vi "Final Tilt Platform Controller.vi"() -> ()   [LabVIEW 2015]
uses:
  Control 1.ctl
  <vilib>/DAQmx/read.llb/DAQmx Read (Analog 1D Wfm NChan NSamp).vi
  <vilib>/DAQmx/read.llb/DAQmx Read (Digital Wfm 1Chan NSamp).vi
  <vilib>/DAQmx/write.llb/DAQmx Write (Digital 1D Bool 1Chan 1Samp).vi
  <vilib>/Utility/file.llb/Read From Spreadsheet File (DBL).vi
  <vilib>/Utility/file.llb/Read Delimited Spreadsheet (DBL).vi
  <vilib>/Utility/file.llb/Write Delimited Spreadsheet (DBL).vi
  <vilib>/DAQmx/create/channels.llb/DAQmx Create Channel (DO-Digital Output).vi
  <vilib>/DAQmx/create/channels.llb/DAQmx Create Channel (AI-Voltage-Basic).vi
  <vilib>/DAQmx/configure/timing.llb/DAQmx Timing (Sample Clock).vi
  <vilib>/DAQmx/configure/trigger.llb/DAQmx Start Trigger (Digital Edge).vi
  <vilib>/DAQmx/create/channels.llb/DAQmx Create Channel (DI-Digital Input).vi
  <vilib>/DAQmx/create/channels.llb/DAQmx Create Channel (CO-Pulse Generation-Ticks).vi
  <vilib>/DAQmx/configure/timing.llb/DAQmx Timing (Implicit).vi
  <vilib>/DAQmx/miscellaneous.llb/DAQmx Fill In Error Info.vi
  <vilib>/Waveform/DTblOps.llb/DTbl Digital to Boolean Array.vi
panel:
  out "incl":dbl[](array[numeric])
  in  "Start from Tilt":i32=1
  out "Ready":bool
  in  "Replay File":path
  in  "Load Sequence":bool
  in  "Format":string="%.3f"
  in  "Delimiter":string=","
  in  "Column/Row Major":bool
  in  "Append to File?":bool=TRUE
  out "File Path":path
  out "Waveform Chart (Multiple Plots)":dbl[][](graph)
  in  "Callib Acce":bool
  in  "Callib Load Cell":bool
  in  "Transect?":bool
  in  "Week Number":dbl
  in  "Rat ID":string
  out "4":bool
  out "5":bool
  out "6":bool
  out "2":bool
  out "1":bool
  out "3":bool
  in  "Baseline Angle":dbl
  out "Angle":i32
  out "Total Force (g)":i32
  out "Completed Tilts":i32
  out "Current Tilt":i32
  out "Current ITI (s)":i32
  in  "Tirgger 6":bool=TRUE
  in  "Enable Left Slow":bool=TRUE
  in  "Enable Left Medium":bool=TRUE
  in  "Enable Left Fast":bool=TRUE
  in  "Enable Right Slow":bool=TRUE
  in  "Enable Right Medium":bool=TRUE
  in  "Enable Right Fast":bool=TRUE
  out "Left Slow":i32
  out "Left Medium":i32
  out "Left Fast":i32
  out "Right Slow":i32
  out "Right Medium":i32
  out "Right Fast":i32
  out "Practice?":bool
  in  "Stop 2":bool
  in  "Pause":bool=TRUE
  in  "Start":bool
  in  "Trial Per Tilt":T1=100.0
  in  "ITI Base (s)":dbl=2.0 format="%#.2g"
  in  "ITI Random Multiplier":dbl=1.0 format="%#.2g"
  in  "Clock Source":i32(slide)=1 caption="Choose a setting:" scale=0.0..1.0
  # "Rat Ground Reaction Forces"
  # "Clock Source"
  # "Tilt Parameters"
  # "Enable"
  # "Animal Info"
  # "Right"
  # "Left"
  # "Current Values"
  # "Enable"
  # "Callibration"
  # "File Information"
  # "Replay Sequence"
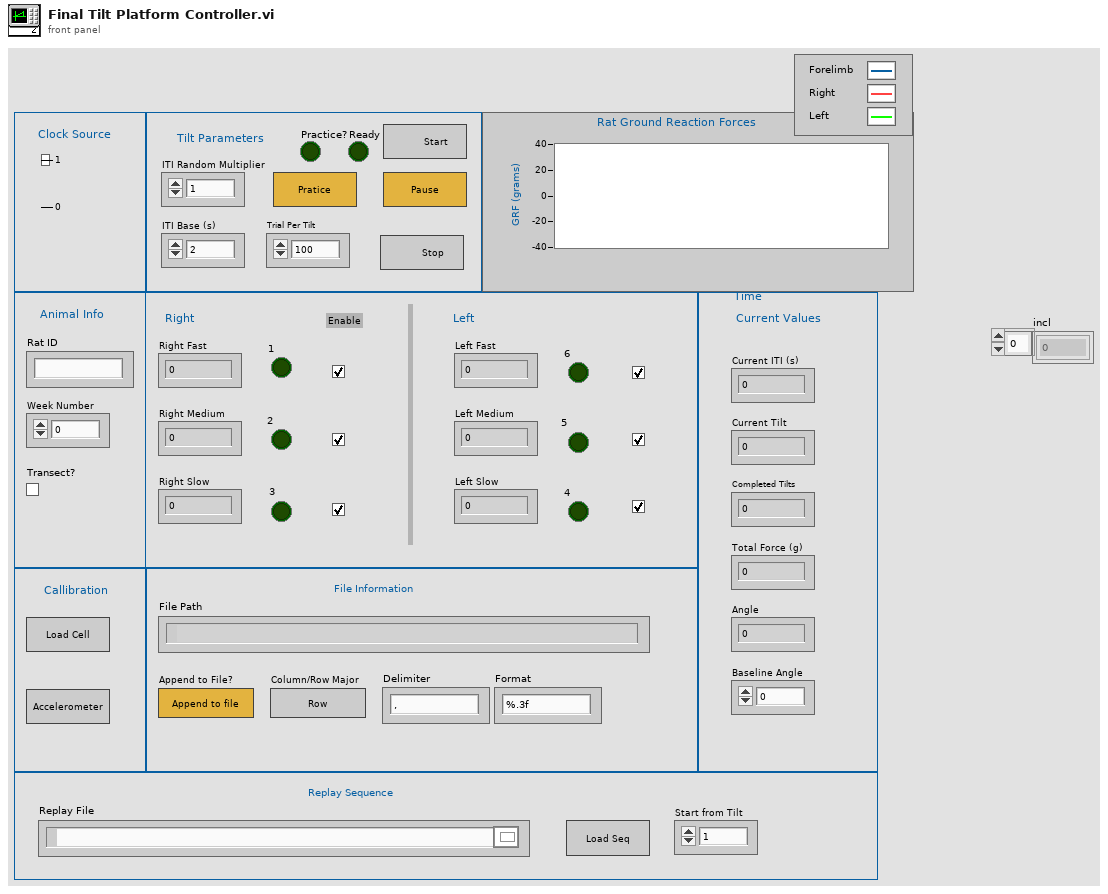
[diagram p1: front panel]
types:
  T1 = typedef "Control 1.ctl" = dbl
  T2 = enum16{"open", "replace", "create", "open or create", "replace or create", "replace or create with confirmation"}
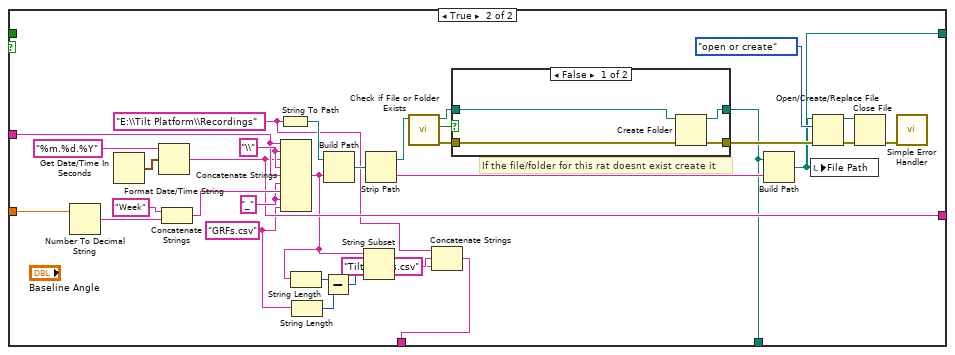
[diagram p2: hidden frame]
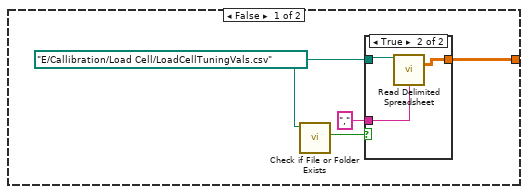
[diagram p4: hidden frame]
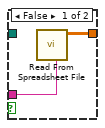
[diagram p5: hidden frame]
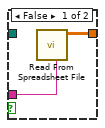
[diagram p6: hidden frame]
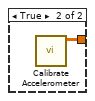
[diagram p7: hidden frame]
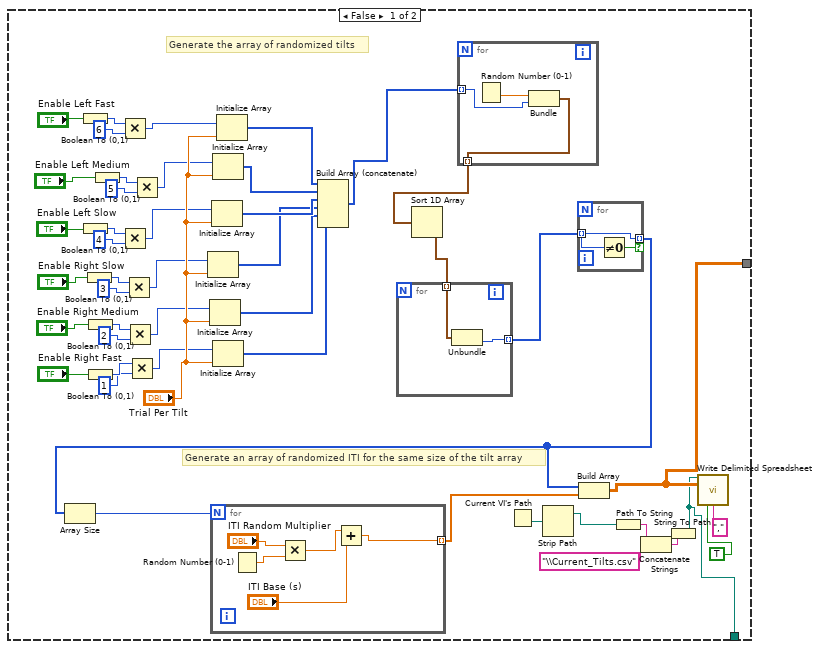
[diagram p8: hidden frame]
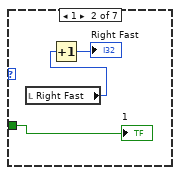
[diagram p12: hidden frame]
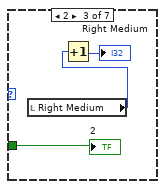
[diagram p13: hidden frame]
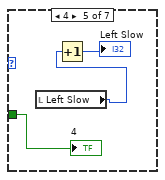
[diagram p14: hidden frame]
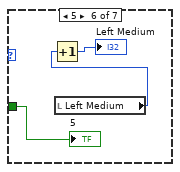
[diagram p15: hidden frame]
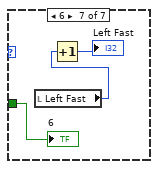
[diagram p16: hidden frame]
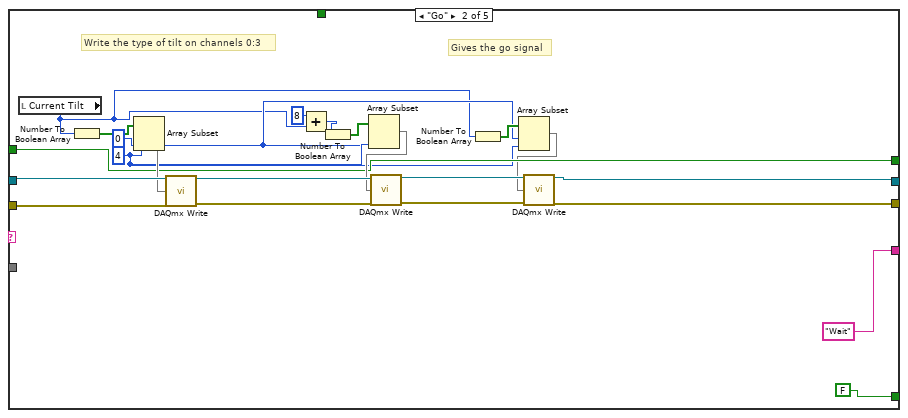
[diagram p17: hidden frame]
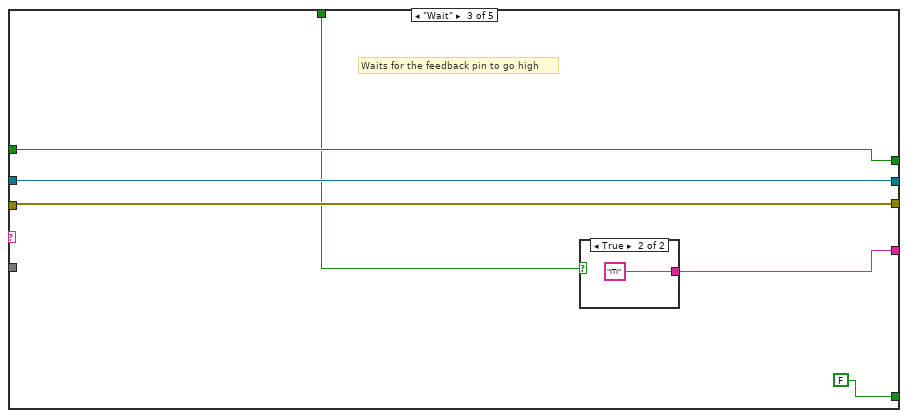
[diagram p18: hidden frame]
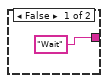
[diagram p19: hidden frame]
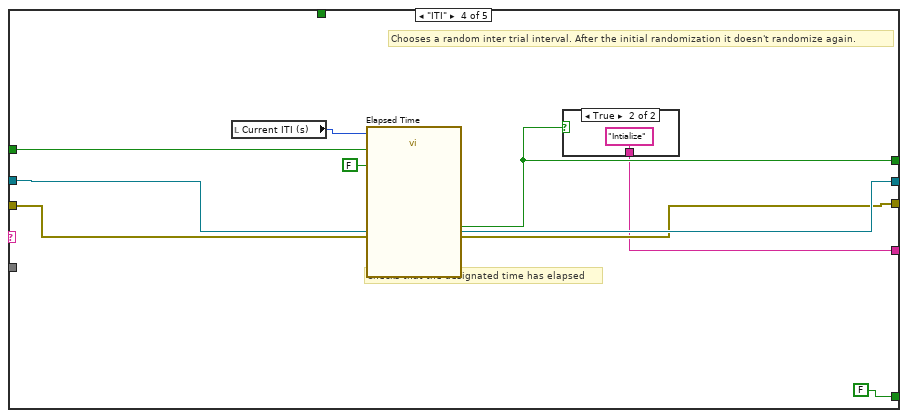
[diagram p20: hidden frame]
diagram:
  # "DataCol/KEY\n1-ai4 (17)=forelimb GRF\n2-ai5 (20)=RHL GRF\n3-ai6 (25)=LHL GRF\n4-ai0=ACC1\n5-ai1=ACC2\n6-ai2=ACC3\n7-ai3=inclinometer"
  # "The GUI these items are not touched. Only through local variables"
  n1 = flat-sequence {
    tunnel: ["Tirgger 6"] -> w70
    tunnel: [w80] -> w69
    tunnel: [w76] -> w63
    tunnel: [w74] -> w15
    tunnel: [w73] -> w8
    tunnel: [w72] -> w1
    tunnel: w70 -> [w127]
    tunnel: [w127] -> w68
    tunnel: w69 -> [w126]
    tunnel: [w126] -> w67
    tunnel: w63 -> [w125]
    tunnel: [w125] -> w62
    tunnel: [w123] -> w30
    tunnel: [w122] -> w16
    tunnel: w15 -> [w122]
    tunnel: [w121] -> w9
    tunnel: w8 -> [w121]
    tunnel: [w120] -> w2
    tunnel: w1 -> [w120]
    tunnel: w68 -> [w146]
    tunnel: [w146] -> w51
    tunnel: [w145] -> w49
    tunnel: w67 -> [w145]
    tunnel: [w144] -> w47
    tunnel: w62 -> [w144]
    tunnel: [w143] -> w31
    tunnel: w30 -> [w143]
    tunnel: [w141] -> w27
    tunnel: [w140] -> w17
    tunnel: w16 -> [w140]
    tunnel: [w139] -> w10
    tunnel: w9 -> [w139]
    tunnel: [w138] -> w3
    tunnel: w2 -> [w138]
    tunnel: w51 -> [w164]
    tunnel: [w164] -> w50
    tunnel: w49 -> [w163]
    tunnel: [w163] -> w48
    tunnel: w47 -> [w162]
    tunnel: [w162] -> w46
    tunnel: [w161] -> w32
    tunnel: w31 -> [w161]
    tunnel: [w160] -> w28
    tunnel: w27 -> [w160]
    tunnel: [w159] -> w18
    tunnel: w17 -> [w159]
    tunnel: [w158] -> w11
    tunnel: w10 -> [w158]
    tunnel: [w157] -> w4
    tunnel: w3 -> [w157]
    tunnel: w50 -> [w175]
    tunnel: [w175] -> w61
    tunnel: w48 -> [w174]
    tunnel: [w174] -> w60
    tunnel: w46 -> [w173]
    tunnel: [w173] -> w59
    tunnel: [w171] -> w45
    tunnel: [w170] -> w33
    tunnel: w32 -> [w170]
    tunnel: w28 -> [w169]
    tunnel: [w169] -> w26
    tunnel: [w168] -> w22
    tunnel: [w167] -> w19
    tunnel: w18 -> [w167]
    tunnel: [w166] -> w12
    tunnel: w11 -> [w166]
    tunnel: [w165] -> w5
    tunnel: w4 -> [w165]
    tunnel: [w301] -> w66
    tunnel: w61 -> [_]
    tunnel: [w294] -> w65
    tunnel: [w293] -> w64
    tunnel: w60 -> [w250]
    tunnel: w59 -> [_]
    tunnel: [w284] -> w58
    tunnel: [w283] -> w57
    tunnel: [w280] -> w52
    tunnel: w45 -> [w279]
    tunnel: [w279] -> w44
    tunnel: [w276] -> w43
    tunnel: [w275] -> w42
    tunnel: [w259] -> w39
    tunnel: [w258] -> w38
    tunnel: w33 -> [w252]
    tunnel: [w252] -> w29
    tunnel: w26 -> [w251]
    tunnel: [w251] -> w25
    tunnel: [w248] -> w23
    tunnel: w22 -> [w248]
    tunnel: [w247] -> w20
    tunnel: w19 -> [w247]
    tunnel: [w246] -> w13
    tunnel: w12 -> [w246]
    tunnel: [w245] -> w6
    tunnel: w5 -> [w245]
    tunnel: w66 -> [w340]
    tunnel: w65 -> [w339]
    tunnel: w64 -> [w337]
    tunnel: w58 -> [w342]
    tunnel: w57 -> [w341]
    tunnel: [w338] -> w56
    tunnel: [w336] -> w55
    tunnel: [w335] -> w54
    tunnel: [w334] -> w53
    tunnel: w52 -> [w332]
    tunnel: w44 -> [w331]
    tunnel: w43 -> [w330]
    tunnel: w42 -> [w329]
    tunnel: [w328] -> w41
    tunnel: [w327] -> w40
    tunnel: w39 -> [w325]
    tunnel: w38 -> [w326]
    tunnel: [w323] -> w37
    tunnel: [w324] -> w36
    tunnel: [w321] -> w35
    tunnel: [w320] -> w34
    tunnel: w29 -> [w319]
    tunnel: w25 -> [w318]
    tunnel: [w317] -> w24
    tunnel: w23 -> [w317]
    tunnel: [w316] -> w21
    tunnel: w20 -> [w316]
    tunnel: [w315] -> w14
    tunnel: w13 -> [w315]
    tunnel: [w314] -> w7
    tunnel: w6 -> [w314]
    tunnel: w56 -> [w522]
    tunnel: w55 -> [w521]
    tunnel: w54 -> [w520]
    tunnel: w53 -> [w519]
    tunnel: w41 -> [w517]
    tunnel: w40 -> [w518]
    tunnel: w37 -> [w512]
    tunnel: w36 -> [w513]
    tunnel: w35 -> [_]
    tunnel: w34 -> [_]
    tunnel: w24 -> [w511]
    tunnel: w21 -> [w510]
    tunnel: w14 -> [w509]
    tunnel: w7 -> [w508]
    frame #0 {
      # "This keeps the program frozen until you hit start. This way it gives you time to change anything you need to update for the tilt types"
      # "Determine if this is a practice session. Causes files not to be saved"
      n2 = while {
        stop <- "Start" stop-if-true
      }
    }
    frame #1 {
      # "If the file doesnt exist create it"
      # "Save the file"
      # "If it's not a practice"
      n3 = Not(x="Tirgger 6") -> (.not. x?=w73:bool)
      n4 = local write "Practice?"("Tirgger 6") -> ()
      n5 = case shown="False" w73 {
        tunnel: "Transect?" -> [_ _]
        tunnel: "Week Number" -> [_ w95]
        tunnel: "Rat ID" -> [_ w94]
        tunnel: [_ w91] -> w80
        tunnel: [_ w93] -> w76
        tunnel: [_ w83] -> w74
        tunnel: [_ w81] -> w72
        frame False {
        }
        frame True {
          w96 = "_"
          w99 = "\\" ("string")
          w84 = "E:\\Tilt Platform\\Recordings"
          w87 = "GRFs.csv" ("string")
          # "If the file/folder for this rat doesnt exist create it"
          n6 = Number To Decimal String(number=w95) -> (decimal integer string=w112:string)  [unwired: 1 in]
          n7 = Get Date/Time In Seconds() -> (seconds since 1Jan1904=w110:timestamp)
          n8 = Format Date/Time String(time format string (%c)="%m.%d.%Y", seconds (now)=w110) -> (date/time string=w93:string)  [unwired: 1 in]
          n9 = Concatenate Strings("Week" ("string"), w112) -> (w98:string)
          n10 = String To Path(string=w84) -> (path=w111:path)
          n11 = Concatenate Strings(w94, w99, w93, w99, w94, w96, w98, w96, w87) -> (w90:string)
          n12 = String Length(string=w90) -> (length=w89:i32)
          n13 = String Length(string=w87) -> (length=w88:i32)
          n14 = Subtract(x=w89, y=w88) -> (x-y=w86:i32)
          n15 = Build Path(base path=w111, name or relative path=w90) -> (appended path=w108:path)
          n16 = String Subset(string=w90, length (rest)=w86) -> (substring=w85:string)  [unwired: 1 in]
          n17 = Strip Path(path=w108) -> (stripped path=w107:path, name=w97:string)
          n18 = call <vilib>:"Check if File or Folder Exists.vi"("path"=w107) -> ("error out"=w105:errorcluster, "file or folder exists?"=w106:bool, "dup path"=w92:path)  [unwired: 8 in]
          n19 = Concatenate Strings(w84, w85, "Tilt_Types.csv" ("string")) -> (w83:string)
          n20 = case shown="False" w106 {
            tunnel: w92 -> [w117 w119]
            tunnel: w105 -> [w116 w118]
            tunnel: [w115 w119] -> w81
            tunnel: [w114 w118] -> w102
            frame False {
              n21 = Create Folder(path (use dialog)=w117, error in=w116) -> (created path=w115:path, error out=w114:errorcluster)  [unwired: 1 in, 1 out]
            }
            frame True {
            }
          }
          n22 = Build Path(base path=w81, name or relative path=w97) -> (appended path=w91:path)
          n23 = local write "File Path"(w91) -> ()
          n24 = Open/Create/Replace File(file path (use dialog)=w91, error in=w102, operation (0:open)=T2."open or create") -> (refnum out=w104:refnum<file>, error out=w101:errorcluster)  [unwired: 3 in, 1 out]
          n25 = Close File(refnum=w104, error in=w101) -> (error out=w100:errorcluster)  [unwired: 1 out]
          n26 = call <vilib>:"Simple Error Handler.vi"("error in (no error)"=w100) -> ()  [unwired: 4 in, 5 out]
        }
      }
    }
    frame #2 {
      # "Otherwise load the previous callibration values"
      # "Pull up sub vi"
      # "If you chose to calibrate the load cells"
      n27 = case shown="True" "Callib Load Cell" {
        tunnel: [w129 w137] -> w123
        frame False {
          w130 = path "E:/Callibration/Load Cell/LoadCellTuningVals.csv" ("file path (dialog if empty)")
          n28 = call <vilib>:"Check if File or Folder Exists.vi"("path"=w130) -> ("file or folder exists?"=w131:bool)  [unwired: 8 in, 2 out]
          n29 = case shown="True" w131 {
            tunnel: w130 -> [_ w135]
            tunnel: [w133 w134] -> w129
            tunnel: "," ("delimiter (\\t)") -> [w132 w136]
            frame False {
              n30 = call-poly <vilib>:"Read From Spreadsheet File.vi"("delimiter (\\t)"=w132) -> ("all rows"=w133:dbl[][])  [unwired: 6 in, 4 out]
            }
            frame True {
              n31 = call-poly <vilib>:"Read Delimited Spreadsheet.vi"("file path (dialog if empty)"=w135, "delimiter (\\t)"=w136) -> ("all rows"=w134:dbl[][])  [unwired: 8 in, 5 out]
            }
          }
        }
        frame True {
          n32 = call "Calibrate load cells.vi"() -> ("Slope and Intercept"=w137:dbl[][])  [unwired: 11 in]
        }
      }
    }
    frame #3 {
      # "Otherwise load the previous values"
      # "Load the sub vi"
      # "If you chose to calibrate the accelerometer"
      n33 = case shown="False" "Callib Acce" {
        tunnel: [w149 w156] -> w141
        frame False {
          w148 = path "E:/Callibration/Accelerometer/AccTuningVals.csv" ("file path (dialog if empty)")
          n34 = call <vilib>:"Check if File or Folder Exists.vi"("path"=w148) -> ("file or folder exists?"=w147:bool)  [unwired: 8 in, 2 out]
          n35 = case shown="True" w147 {
            tunnel: "," ("delimiter (\\t)") -> [w151 w155]
            tunnel: [w152 w154] -> w149
            tunnel: w148 -> [_ w153]
            frame False {
              n36 = call-poly <vilib>:"Read From Spreadsheet File.vi"("delimiter (\\t)"=w151) -> ("all rows"=w152:dbl[][])  [unwired: 6 in, 4 out]
            }
            frame True {
              n37 = call-poly <vilib>:"Read Delimited Spreadsheet.vi"("file path (dialog if empty)"=w153, "delimiter (\\t)"=w155) -> ("all rows"=w154:dbl[][])  [unwired: 8 in, 5 out]
            }
          }
        }
        frame True {
          n38 = call "Calibrate Accelerometer.vi"() -> ("Output"=w156:dbl[][])  [unwired: 9 in]
        }
      }
    }
    frame #4 {
    }
    frame #5 {
      # "Is this a practice session?"
      # "load cell regression params"
      # "acceleremeter regression params"
      n39 = case shown="True" "Load Sequence" {
        tunnel: [w177 w235] -> w171
        tunnel: [w176 _] -> w168
        frame False {
          # "Generate an array of randomized ITI for the same size of the tilt array"
          # "Generate the array of randomized tilts"
          n40 = Boolean To (0,1)(Boolean="Enable Left Fast") -> (0, 1=w219:i16)
          n41 = Boolean To (0,1)(Boolean="Enable Left Slow") -> (0, 1=w211:i16)
          n42 = Boolean To (0,1)(Boolean="Enable Right Slow") -> (0, 1=w208:i16)
          n43 = Boolean To (0,1)(Boolean="Enable Right Medium") -> (0, 1=w203:i16)
          n44 = Boolean To (0,1)(Boolean="Enable Right Fast") -> (0, 1=w199:i16)
          n45 = Boolean To (0,1)(Boolean="Enable Left Medium") -> (0, 1=w216:i16)
          n46 = Multiply(x=w219, y=6 ("length")) -> (x*y=w213:i32)
          n47 = Multiply(x=w211, y=4 ("length")) -> (x*y=w205:i32)
          n48 = Multiply(x=w208, y=3 ("length")) -> (x*y=w204:i32)
          n49 = Multiply(x=w203, y=2 ("length")) -> (x*y=w200:i32)
          n50 = Multiply(x=w199, y=1 ("length")) -> (x*y=w196:i32)
          n51 = Multiply(x=w216, y=5 ("length")) -> (x*y=w212:i32)
          n52 = Initialize Array(w204, "Trial Per Tilt") -> (w192:i32[])
          n53 = Initialize Array(w200, "Trial Per Tilt") -> (w191:i32[])
          n54 = Initialize Array(w205, "Trial Per Tilt") -> (w193:i32[])
          n55 = Initialize Array(w212, "Trial Per Tilt") -> (w194:i32[])
          n56 = Initialize Array(w196, "Trial Per Tilt") -> (w190:i32[])
          n57 = Initialize Array(w213, "Trial Per Tilt") -> (w195:i32[])
          n58 = Build Array (concatenate)(w195, w194, w193, w192, w191, w190) -> (w188:i32[])
          n59 = for {
            tunnel: w188 -> [w232] mode=indexing
            tunnel: [w233] -> w222 mode=indexing
            n60 = Random Number (0-1)() -> (number: 0 to 1=w234:dbl)
            n61 = Bundle("number: 0 to 1"=w234, w232) -> (w233:cluster{"number: 0 to 1":dbl, i32})  [unwired: 1 in]
          }
          n62 = Sort 1D Array(array=w222) -> (sorted array=w221:cluster{"number: 0 to 1":dbl, i32}[])
          n63 = for {
            tunnel: w221 -> [w231] mode=indexing
            tunnel: [w230] -> w189 mode=indexing
            n64 = Unbundle(w231) -> (w230:i32)  [unwired: 1 out]
          }
          n65 = Current VI's Path() -> (path=w184:path)
          n66 = Strip Path(path=w184) -> (stripped path=w183:path)  [unwired: 1 out]
          n67 = for {
            tunnel: [w228] -> w178 mode=indexing if=w229
            tunnel: w189 -> [w228] mode=indexing
            n68 = Not Equal To 0?(x=w228) -> (x != 0?=w229:bool)
          }
          n69 = Array Size(array=w178) -> (size(s)=w187:i32)
          n70 = for {
            N: w187 -> [_]
            tunnel: [w223] -> w186 mode=indexing
            n71 = Random Number (0-1)() -> (number: 0 to 1=w226:dbl)
            n72 = Multiply(x="ITI Random Multiplier", y=w226) -> (x*y=w225:dbl)
            n73 = Add(x=w225, y="ITI Base (s)") -> (x+y=w223:dbl)
          }
          n74 = Build Array(w178, w186) -> (w177:dbl[][])
          n75 = Path To String(path=w183) -> (string=w182:string)
          n76 = Concatenate Strings(w182, "\\Current_Tilts.csv") -> (w180:string)
          n77 = String To Path(string=w180) -> (path=w176:path)
          n78 = call-poly <vilib>:"Write Delimited Spreadsheet.vi"("file path (dialog if empty)"=w176, "2D data"=w177, "transpose? (F)"=TRUE ("transpose? (no:F)"), "delimiter (\\t)"="," ("delimiter (\\t)")) -> ()  [unwired: 10 in, 2 out]
        }
        frame True {
          n79 = Decrement(x="Start from Tilt") -> (x-1=w237:i32)
          n80 = call-poly <vilib>:"Read Delimited Spreadsheet.vi"("file path (dialog if empty)"="Replay File", "delimiter (\\t)"="," ("delimiter (\\t)")) -> ("all rows"=w242:dbl[][])  [unwired: 8 in, 5 out]
          n81 = Array Size(array=w242) -> (size(s)=w241:i32[])
          n82 = Array Max & Min(array=w241) -> (max value=w239:i32)  [unwired: 3 out]
          n83 = Subtract(x=w239, y=w237) -> (x-y=w240:i32)
          n84 = Array Subset(array=w242, index (row)=w237, length (row)=w240) -> (w236:dbl[][])  [unwired: 2 in]
          n85 = Transpose 2D Array(2D array=w236) -> (transposed array=w235:dbl[][])
        }
      }
    }
    frame #6 {
      w263 = 10214 items=["High"=10192, "Low"=10214] ("idle state")
      w262 = 10123 items=["Finite Samples"=10178, "Continuous Samples"=10123, "Hardware Timed Single Point"=12522] ("sample mode")
      w281 = 10123 items=["Finite Samples"=10178, "Continuous Samples"=10123, "Hardware Timed Single Point"=12522] ("sample mode")
      w295 = 10083 items=["default"=-1, "RSE"=10083, "NRSE"=10078, "Differential"=10106, "Pseudodifferential"=12529] ("input terminal configuration")
      w287 = 1000.0 ("rate")
      # "Filename for data file"
      # "A 2D array of tilts and ITIs from a file or generated just now"
      # "Merging the errors for  digital and analog input tasks"
      # "Using analog sample clock to get digital data"
      # "change back to 16"
      # "This is the repeated sequence array"
      n86 = Array Size(array=w279) -> (size(s)=w292:i32[])
      n87 = Greater?(x=w292, y=0) -> (0:w278:bool[])
      n88 = And Array Elements(Boolean array=w278) -> (logical AND=→"Ready":bool)
      n89 = Subtract(x=u32 40 ("Divisor"), y=u32 2 ("high ticks")) -> (x-y=w271:u32)
      n90 = case shown="0" "Clock Source" {
        tunnel: [_ tag "/Dev3/PFI2" ("source")] -> w272
        frame 1, Default {
        }
        frame 0 {
        }
      }
      n91 = call-poly <vilib>:"DAQmx Create Virtual Channel.vi"("high ticks"=u32 2, "low ticks"=w271, "counter"=tag "Dev3/ctr0" ("Counter to Use"), "source of ticks"=tag "/Dev3/PFI0" ("Signal Input"), "idle state"=w263, "initial delay"=w271) -> ("task out"=w264:refnum<k21>, "error out"=w265:errorcluster)  [unwired: 8 in]
      n92 = call-poly <vilib>:"DAQmx Create Virtual Channel.vi"("lines"=tag "Dev3/port0/line4") -> ("task out"=w288:refnum<k21>, "error out"=w289:errorcluster)  [unwired: 13 in]
      n93 = call-poly <vilib>:"DAQmx Create Virtual Channel.vi"("maximum value"=10.0, "minimum value"=-10.0, "input terminal configuration"=w295, "physical channels"=tag "Dev3/ai4:6,Dev3/ai0:2,Dev3/ai3") -> ("task out"=w296:refnum<k21>, "error out"=w297:errorcluster)  [unwired: 10 in]
      n94 = call-poly <vilib>:"DAQmx Timing.vi"("task/channels in"=w264, "sample mode"=w262, "error in"=w265) -> ("task out"=w260:refnum<k21>, "error out"=w261:errorcluster)  [unwired: 11 in]
      n95 = call-poly <vilib>:"DAQmx Timing.vi"("task/channels in"=w288, "sample mode"=w281, "rate"=w287, "source"=tag "/Dev3/ai/SampleClock", "error in"=w289) -> ("task out"=w286:refnum<k21>, "error out"=w285:errorcluster)  [unwired: 9 in]
      n96 = call-poly <vilib>:"DAQmx Timing.vi"("task/channels in"=w296, "sample mode"=w281, "rate"=w287, "source"=w272, "error in"=w297) -> ("task out"=w257:refnum<k21>, "error out"=w255:errorcluster)  [unwired: 9 in]
      n97 = call <vilib>:"DAQmx Start Task.vi"("task/channels in"=w260, "error in"=w261) -> ("task out"=w259:refnum<k21>, "error out"=w258:errorcluster)  [unwired: 12 in]
      n98 = call <vilib>:"DAQmx Start Task.vi"("task/channels in"=w286, "error in"=w285) -> ("task out"=w283:refnum<k21>, "error out"=w284:errorcluster)  [unwired: 12 in]
      n99 = case shown="0" "Clock Source" {
        tunnel: w257 -> [w306 w312]
        tunnel: [w306 w311] -> w256
        tunnel: w255 -> [w305 w310]
        tunnel: [w305 w309] -> w254
        frame 1, Default {
        }
        frame 0 {
          w308 = 10171 items=["Rising"=10280, "Falling"=10171] ("edge")
          n100 = call-poly <vilib>:"DAQmx Trigger.vi"("task/channels in"=w312, "source"=tag "/Dev3/PFI1", "edge"=w308, "error in"=w310) -> ("task out"=w311:refnum<k21>, "error out"=w309:errorcluster)  [unwired: 10 in]
        }
      }
      n101 = call-poly <vilib>:"DAQmx Create Virtual Channel.vi"("lines"=tag "Dev3/port0/line0:3") -> ("task out"=w303:refnum<k21>, "error out"=w302:errorcluster)  [unwired: 13 in]
      n102 = Merge Errors(w258, w254, w284) -> (w282:errorcluster)
      n103 = call <vilib>:"DAQmx Start Task.vi"("task/channels in"=w303, "error in"=w302) -> ("task out"=w301:refnum<k21>, "error out"=w280:errorcluster)  [unwired: 12 in]
      n104 = Open/Create/Replace File(file path (use dialog)=w250, operation (0:open)=T2."open or create", access (0:read/write)=enum16{"read/write", "read-only", "write-only"}."write-only") -> (refnum out=w276:refnum<file>, error out=w275:errorcluster)  [unwired: 3 in, 1 out]
      n105 = call <vilib>:"DAQmx Start Task.vi"("task/channels in"=w256, "error in"=w282) -> ("task out"=w294:refnum<k21>, "error out"=w293:errorcluster)  [unwired: 12 in]
    }
    frame #7 {
      # "Start the state machine with \"intialize\""
      n106 = while {
        tunnel: w342 -> [w412]
        tunnel: w341 -> [w417]
        tunnel: w340 -> [w408]
        tunnel: w332 -> [w407]
        tunnel: [w416] -> w338
        tunnel: w339 -> [w418]
        tunnel: w337 -> [w415]
        tunnel: [w414] -> w336
        tunnel: [w413] -> w335
        tunnel: [w383] -> w334
        shift-right: [w409] -> _
        shift-left: " Intialize" -> [w410]
        shift-right: [w406] -> _
        shift-left: TRUE ("Time has Elapsed") -> [w405]
        tunnel: w331 -> [w402]
        tunnel: w330 -> [w373]
        tunnel: w329 -> [w372]
        tunnel: [w382] -> w328
        tunnel: [w381] -> w327
        tunnel: w326 -> [w380]
        tunnel: w325 -> [w379]
        tunnel: [w378] -> w323
        tunnel: [w377] -> w324
        tunnel: [w370] -> w321
        tunnel: [w369] -> w320
        tunnel: w319 -> [w368]
        tunnel: w318 -> [w343]
        stop <- w404 stop-if-true
        (unwired) FALSE ("prepend array or string size? (T)")
        # "saving the raw accelerometer data"
        # "accelerometer params"
        # "Load cell params"
        # "Plot only load cells"
        # "convert all the waveforms read into a data array then convert into string to write to file"
        # "Use an OR statement to concatinate the 10 digital signals read"
        # "Read in 10 samples per iteration for both analog and digital data"
        # "The program can only end if its we're in the intialize stage"
        # "Currrent state"
        # "Reset for ITI timer"
        # "Feedback from motor signalling tilt complete"
        # "Current Tilt"
        # "Update the count for a given tilt type"
        # "Right Fast = 1\nRight Mid = 2\nRight Slow = 3\nLeft Fast = 4\nLeft Mid = 5\nLeft Slow = 6"
        # "Stops the loop"
        # "Digital input"
        # "Analog input"
        # "Digital output"
        n107 = call-poly <vilib>:"DAQmx Read.vi"("task/channels in"=w418, "number of samples per channel"=100, "error in"=w415) -> ("task out"=w416:refnum<k21>, "data"=w357:waveform(dbl)[], "error out"=w414:errorcluster)  [unwired: 10 in]
        n108 = call-poly <vilib>:"DAQmx Read.vi"("task/channels in"=w417, "number of samples per channel"=100, "error in"=w412) -> ("task out"=w413:refnum<k21>, "data"=w375:digitalwaveform, "error out"=w383:errorcluster)  [unwired: 10 in]
        n109 = Unbundle By Name(w375) -> ("Y"=w365:digitaldata)
        n110 = call <vilib>:"DAQmx Is Task Done.vi"("task/channels in"=w379, "error in"=w380) -> ("task out"=w378:refnum<k21>, "error out"=w377:errorcluster)  [unwired: 11 in, 1 out]
        n111 = call-poly <vilib>:"Digital to Boolean Array.vi"("digital data"=w365) -> ("boolean array"=w367:bool[][])  [unwired: 9 in, 1 out]
        n112 = And Array Elements(Boolean array=w367) -> (logical AND=w374:bool)
        n113 = case shown="\"Choose Tilt\"" w410 {
          tunnel: ["Go" "Wait" w476 w484 w504] -> w409
          tunnel: w408 -> [w431 w471 w478 w487 w503]
          tunnel: w407 -> [w430 w470 w477 w486 w502]
          tunnel: [w431 w460 w478 w487 w503] -> w382
          tunnel: [w430 w459 w477 w486 w502] -> w381
          tunnel: [w429 w463 w475 w485 w501] -> w406
          tunnel: w405 -> [w429 w463 w475 w483 w501]
          tunnel: [FALSE FALSE FALSE FALSE TRUE] -> w403
          tunnel: w402 -> [w426 _ _ _ w499]
          tunnel: w374 -> [_ _ w473 _ _]
          frame "Choose Tilt" {
            # "Turn on the LED for the chosen tilt"
            # "Update the current ITI and tilt values"
            # "This has just one Tilt and ITI"
            # "We select the top most index from the array"
            # "This array has the tilt & ITI"
            # "Build an array where the disabled tilt types are set to zero"
            n114 = local read "Completed Tilts"() -> (w419:i32)
            n115 = Index Array(array=w426, index (col)=w419) -> (element=w425:dbl[])  [unwired: 1 in]
            n116 = Index Array(array=w425, index #1=0 ("index"), index #2=1 ("index")) -> (element #1=w422:dbl, element #2=→"Current ITI (s)":dbl)
            "Current Tilt" <- w422
            n117 = Increment(x=w419) -> (x+1=→"Completed Tilts":i32)
            n118 = case shown="3" w422 {
              tunnel: TRUE -> [_ w433 w436 w439 w442 w445 w448]
              frame Default {
              }
              frame 1 {
                n119 = local read "Right Fast"() -> (w434:i32)
                n120 = Increment(x=w434) -> (x+1=→"Right Fast":i32)
                "1" <- w433
              }
              frame 2 {
                n121 = local read "Right Medium"() -> (w437:i32)
                n122 = Increment(x=w437) -> (x+1=→"Right Medium":i32)
                "2" <- w436
              }
              frame 3 {
                n123 = local read "Right Slow"() -> (w440:i32)
                n124 = Increment(x=w440) -> (x+1=→"Right Slow":i32)
                "3" <- w439
              }
              frame 4 {
                n125 = local read "Left Slow"() -> (w443:i32)
                n126 = Increment(x=w443) -> (x+1=→"Left Slow":i32)
                "4" <- w442
              }
              frame 5 {
                n127 = local read "Left Medium"() -> (w446:i32)
                n128 = Increment(x=w446) -> (x+1=→"Left Medium":i32)
                "5" <- w445
              }
              frame 6 {
                n129 = local read "Left Fast"() -> (w449:i32)
                n130 = Increment(x=w449) -> (x+1=→"Left Fast":i32)
                "6" <- w448
              }
            }
          }
          frame "Go" {
            w453 = 4 ("length")
            w452 = 0 ("index")
            # "Gives the go signal"
            # "Write the type of tilt on channels 0:3"
            n131 = local read "Current Tilt"() -> (w451:i32)
            n132 = Number To Boolean Array(number=w451) -> (Boolean array=w467:bool[])
            n133 = Array Subset(array=w467, index=w452, length=w453) -> (w466:bool[])
            n134 = call-poly <vilib>:"DAQmx Write.vi"("task/channels in"=w471, "data"=w466, "error in"=w470) -> ("task out"=w469:refnum<k21>, "error out"=w468:errorcluster)  [unwired: 10 in, 1 out]
            n135 = Add(x=u8 8, y=w451) -> (x+y=w455:i32)
            n136 = Number To Boolean Array(number=w455) -> (Boolean array=w465:bool[])
            n137 = Array Subset(array=w465, index=w452, length=w453) -> (w464:bool[])
            n138 = call-poly <vilib>:"DAQmx Write.vi"("task/channels in"=w469, "data"=w464, "error in"=w468) -> ("task out"=w462:refnum<k21>, "error out"=w461:errorcluster)  [unwired: 10 in, 1 out]
            n139 = Number To Boolean Array(number=w451) -> (Boolean array=w458:bool[])
            n140 = Array Subset(array=w458, index=w452, length=w453) -> (w457:bool[])
            n141 = call-poly <vilib>:"DAQmx Write.vi"("task/channels in"=w462, "data"=w457, "error in"=w461) -> ("task out"=w460:refnum<k21>, "error out"=w459:errorcluster)  [unwired: 10 in, 1 out]
          }
          frame "Wait" {
            # "Waits for the feedback pin to go high"
            n142 = case shown="True" w473 {
              tunnel: ["Wait" "ITI"] -> w476
              frame False {
              }
              frame True {
              }
            }
          }
          frame "ITI" {
            # "Checks that the designated time has elapsed"
            # "Chooses a random inter trial interval. After the initial randomization it doesn't randomize again."
            n143 = local read "Current ITI (s)"() -> (w481:i32)
            n144 = call "Elapsed Time"("Time Target (s)"=w481, "Reset"=w483, "Auto Reset"=FALSE) -> ("Time has Elapsed"=w485:bool)  [unwired: 9 in, 7 out]
            n145 = case shown="True" w485 {
              tunnel: ["ITI" "Intialize"] -> w484
              frame False {
              }
              frame True {
              }
            }
          }
          frame "Intialize", Default {
            w505 = FALSE
            n146 = local write "1"(w505) -> ()
            n147 = local write "2"(w505) -> ()
            n148 = local write "3"(w505) -> ()
            n149 = Array Size(array=w499) -> (size(s)=w498:i32[])
            n150 = local write "4"(w505) -> ()
            n151 = local write "6"(w505) -> ()
            n152 = local write "5"(w505) -> ()
            n153 = Index Array(array=w498, index=1) -> (element=w496:i32)
            n154 = local read "Completed Tilts"() -> (w495:i32)
            n155 = Greater Or Equal?(x=w495, y=w496) -> (x >= y?=w493:bool)
            n156 = Or(x="Pause", y=w493) -> (x .or. y?=w494:bool)
            n157 = Not(x=w494) -> (.not. x?=w492:bool)
            n158 = case shown="False" w492 {
              tunnel: ["Intialize" "Choose Tilt"] -> w504
              frame False {
              }
              frame True {
              }
            }
          }
        }
        n159 = Index Array(array=w357, index #1=0 ("number of samples per channel"), index #2=1 ("number of samples per channel"), index #3=2 ("number of samples per channel"), index #4=3 ("number of samples per channel"), index #5=4 ("number of samples per channel"), index #6=5 ("number of samples per channel"), index #7=6 ("number of samples per channel")) -> (element #1=w394:waveform(dbl), element #2=w393:waveform(dbl), element #3=w392:waveform(dbl), element #4=w391:waveform(dbl), element #5=w390:waveform(dbl), element #6=w389:waveform(dbl), element #7=w388:waveform(dbl))
        n160 = Unbundle By Name(w393) -> ("Y"=w351:dbl[])
        n161 = Unbundle By Name(w392) -> ("Y"=w350:dbl[])
        n162 = Unbundle By Name(w391) -> ("Y"=w346:dbl[])
        n163 = Unbundle By Name(w390) -> ("Y"=w345:dbl[])
        n164 = Unbundle By Name(w394) -> ("Y"=w352:dbl[])
        n165 = Unbundle By Name(w389) -> ("Y"=w344:dbl[])
        n166 = Unbundle By Name(w388) -> ("Y"=w353:dbl[])
        n167 = call "Linear Regression for Load Cell.vi"("x3"=w350, "x2"=w351, "X1"=w352, "slope-intercept"=w368) -> ("Force HL"=w347:dbl[], "Force HR"=w348:dbl[], "Force Forepaw"=w349:dbl[])  [unwired: 5 in]
        n168 = Build Array(w349, w348, w347) -> (w356:dbl[][])
        n169 = Transpose 2D Array(2D array=w356) -> (transposed array=→"Waveform Chart (Multiple Plots)":dbl[][])
        n170 = Boolean To (0,1)(Boolean=w367) -> (0, 1=w366:i16[][])
        n171 = Reshape Array(w366, 1 ("dimension size")) -> (w354:i16[])
        n172 = Build Array(w349, w348, w347, w346, w345, w344, w353, w354) -> (w385:dbl[][])
        n173 = Multiply(x=w353, y=1.834) -> (x*y=w362:dbl[])
        n174 = Transpose 2D Array(2D array=w385) -> (transposed array=w384:dbl[][])
        n175 = Subtract(x=w362, y=2.458) -> (x-y=w360:dbl[])
        n176 = Array To Spreadsheet String(delimiter (Tab)=",", array=w384, 3:"%3f" ("format string")) -> (spreadsheet string=w371:string)
        n177 = Write to Text File(file (use dialog)=w373, text=w371, error in=w372) -> (refnum out=w370:refnum<file>, error out=w369:errorcluster)  [unwired: 1 in, 1 out]
        n178 = Divide(x=w360, y=0.01677) -> (x/y=→"incl":dbl[])
        n179 = call "Determine Acc Angle.vi"("za"=w344, "ya"=w345, "xa"=w346, "Acc"=w343) -> ()  [unwired: 4 in, 4 out]
        n180 = local read "Stop 2"() -> (w404:bool)
        n181 = And(x=w403, y=w404) -> ()  [unwired: 1 out]
      }
    }
    frame #8 {
      # "Clear digital ouput tasks"
      # "accelerometer regression params"
      # "Perform post processing here:"
      # "Clear digital input task"
      # "Clear analog input task"
      # "Clear digital output task"
      # "Resets all values once program ends"
      n182 = case shown="True" w509 {
        tunnel: w511 -> [_ w529]
        tunnel: w510 -> [_ w528]
        tunnel: w508 -> [_ w527]
        frame False {
        }
        frame True {
          n183 = String To Path(string=w528) -> ()  [unwired: 1 out]
          n184 = Move(source path=w529, 9:TRUE ("overwrite (F)"), 10:w527) -> ()  [unwired: 2 in, 3 out]
        }
      }
      n185 = call <vilib>:"DAQmx Clear Task.vi"("task in"=w520, "error in"=w519) -> ()  [unwired: 13 in, 1 out]
      n186 = call <vilib>:"DAQmx Clear Task.vi"("task in"=w517, "error in"=w518) -> ()  [unwired: 13 in, 1 out]
      n187 = call <vilib>:"DAQmx Clear Task.vi"("task in"=w522, "error in"=w521) -> ()  [unwired: 13 in, 1 out]
      n188 = call <vilib>:"DAQmx Stop Task.vi"("task/channels in"=w512, "error in"=w513) -> ("task out"=w516:refnum<k21>, "error out"=w515:errorcluster)  [unwired: 12 in]
      n189 = call <vilib>:"DAQmx Clear Task.vi"("task in"=w516, "error in"=w515) -> ("error out"=w514:errorcluster)  [unwired: 13 in]
      n190 = call <vilib>:"Simple Error Handler.vi"("error in (no error)"=w514) -> ()  [unwired: 4 in, 5 out]
      n191 = control-ref of="This VI"() -> (w525:refnum<vi>)
      n192 = invoke class="VI" method="Default Vals.Reinit All"(reference=w525) -> (reference out=w523:refnum<vi>, error out=w524:errorcluster)  [unwired: 2 in, 1 out]
      n193 = Close Reference(reference=w523, error in (no error)=w524) -> ()  [unwired: 1 out]
    }
  }
